vi "Tdms.Group.Filter.vi"(8 "error in (no error)":errorcluster, 10 "filter string":string, 11 "Refnum in":refnum<k34>) -> (0 "error out":errorcluster, 2 "Array":string[](array[string]), 3 "Refnum out":refnum<k34>)   [LabVIEW 2013]
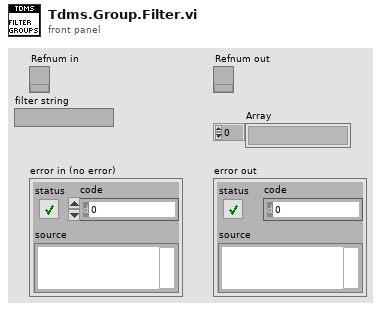
[diagram p1: front panel]
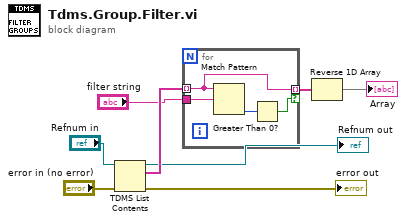
[diagram p0: block diagram]
diagram:
  n1 = TDMS List Contents(4:"error in (no error)", 7:"Refnum in") -> (0:→"error out":errorcluster, 2:w8:string[], 3:→"Refnum out":refnum<k34>)  [unwired: 1 in, 1 out]
  n2 = for {
    tunnel: "filter string" -> [w12]
    tunnel: w8 -> [w10] mode=indexing
    tunnel: [w10] -> w7 mode=indexing if=w9
    n3 = Match Pattern(string=w10, regular expression=w12) -> (offset past match=w11:i32)  [unwired: 1 in, 3 out]
    n4 = Greater Than 0?(x=w11) -> (x > 0?=w9:bool)
  }
  n5 = Reverse 1D Array(array=w7) -> (reversed array=→"Array":string[])
